vi "Live window-Refresh graphs.vi"(9 "Right Channel":T2, 10 "Left Channel":T2, 11 "Element to queue":T3) -> (0 "Right image":T1, 1 "Enable right image":bool, 2 "Enable left image":bool, 3 "Left image":T1)   [LabVIEW 2013]
uses:
  Queue/Live graphs queue/Typedefs/Live imaging queue element.ctl
  <vilib>/vision/Image Controls.llb/IMAQ Image.ctl
  Typedefs/Channel Selector.ctl
  Typedefs/Left-Right enum.ctl
  Global Variables/gl_UI Ctrl Refs.vi
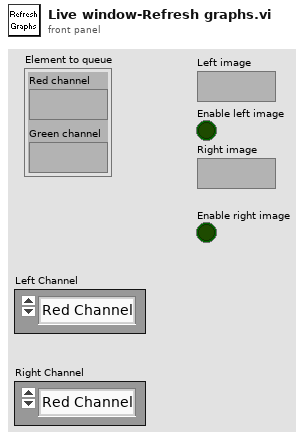
[diagram p1: front panel]
types:
  T1 = typedef "IMAQ Image.ctl" = refnum<image>
  T2 = typedef "Channel Selector.ctl" = enum16{"Red Channel", "Green Channel", "Blended"}
  T3 = typedef "Live imaging queue element.ctl" = cluster{"Red channel":T1, "Green channel":T1}
  T4 = typedef "Left-Right enum.ctl" = enum16{"Right", "Left"}
  T5 = typedef "UI ctrl refs cluster.ctl" = cluster{"Top level VI path":path, "Top level VI ref":refnum<vi>, "User menu ref":refnum<k9>, "Sub Panel control":refnum<vi>, "Imaging Param Tab":refnum<vi>, "Occurrence-Start drivers":refnum<k4>, "Occurrence-Speed logging initialised":refnum<k4>, "Occurrence-XYZ stage initialised":refnum<k4>, "Exit button":refnum<vi>, "Status ind":refnum<vi>, "Return to Origin":refnum<vi>, "Speed Logging":refnum<vi>, "Time Lapse":refnum<vi>, "Live Imaging":refnum<vi>, "AOL Z Stack":refnum<vi>, "Motor Z Stack":refnum<vi>, "Funct Acq button":refnum<vi>, "Hard Shutter":refnum<vi>, "Virtual Shutter":refnum<vi>, "Laser Power":refnum<vi>, "AOL Mode":refnum<vi>, "Frame Size":refnum<vi>, "Field of View":refnum<vi>, "Dwell Time":refnum<vi>, "Zoom":refnum<vi>, "AOL Z":refnum<vi>, "Objective":refnum<vi>, "Axis":refnum<vi>, "Paths & Names":refnum<vi>, "Experiment folder path (ind.)":refnum<vi>, "Last State (Ind.)":refnum<vi>, "Laser wavelength ind (nm)":refnum<vi>, "Averages":refnum<vi>, "Angle (degrees)":refnum<vi>, "X centre":refnum<vi>, "Y centre":refnum<vi>, "Plane Mode":refnum<vi>, "# Planes":refnum<vi>, "Z Start":refnum<vi>, "Z Stop":refnum<vi>, "Z Step":refnum<vi>, "PMT 1":refnum<vi>, "PMT 2":refnum<vi>, "Stage XYZ Position":refnum<vi>, "Pockels@Z Start":refnum<vi>, "Pockels@Z Stop":refnum<vi>, "Obtain Z Start":refnum<vi>, "Obtain Z Stop":refnum<vi>, "Live stim.trig.period":refnum<vi>, "Live stim.trig.enable":refnum<vi>, "Funct. Acq. Pockels Modulation":refnum<vi>, "Enable Video Recording":refnum<vi>, "Video Record-Live Imaging":refnum<vi>, "Video Record-Funct acq":refnum<vi>, "AOL Z-stack Chirps Ready (ind)":refnum<vi>, "Center freq ind (nm)":refnum<vi>, "Logging queue (ind)":refnum<vi>, "Back aperture power (ind.)":refnum<vi>, "Power after objective (ind.)":refnum<vi>, "Switch user":refnum<vi>}
  T6 = typedef "PMT control knob.ctl" = u16
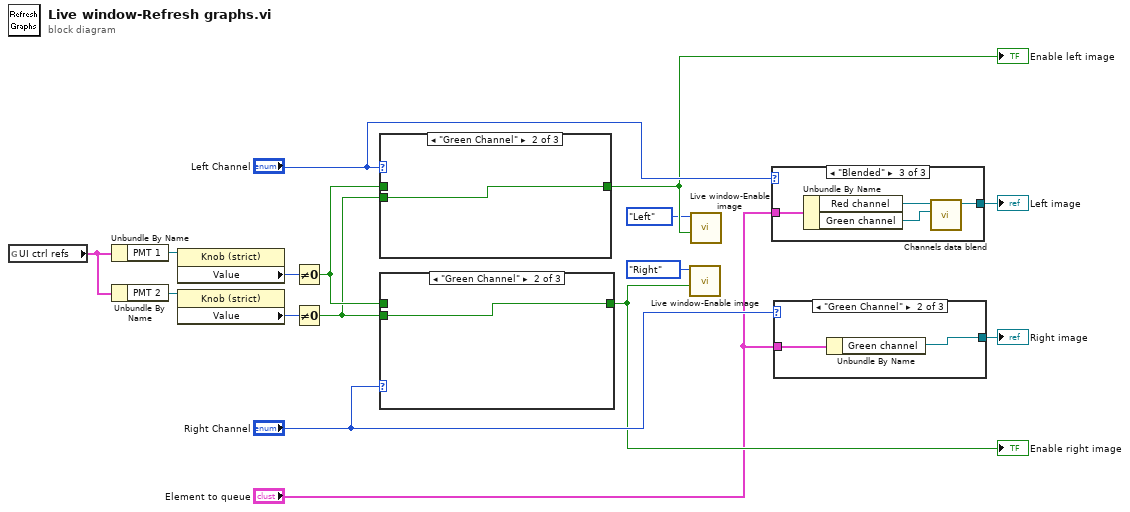
[diagram p0: block diagram]
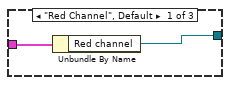
[diagram p2: hidden frame]
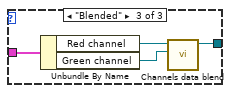
[diagram p3: hidden frame]
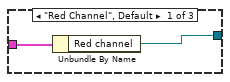
[diagram p4: hidden frame]
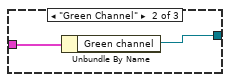
[diagram p5: hidden frame]
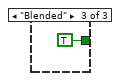
[diagram p7: hidden frame]
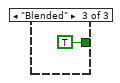
[diagram p9: hidden frame]
diagram:
  n1 = global read "gl_UI Ctrl Refs.vi" "UI ctrl refs"() -> (w12:T5)
  n2 = Unbundle By Name(w12) -> ("PMT 1"=w14:refnum<vi>)
  n3 = Unbundle By Name(w12) -> ("PMT 2"=w13:refnum<vi>)
  n4 = property on="Property Node" class="Knob (strict)"(reference=w14) -> ("Value"=w11:T6)  [unwired: 1 in, 2 out]
  n5 = property on="Property Node" class="Knob (strict)"(reference=w13) -> ("Value"=w10:T6)  [unwired: 1 in, 2 out]
  n6 = Not Equal To 0?(x=w11) -> (x != 0?=w5:bool)
  n7 = Not Equal To 0?(x=w10) -> (x != 0?=w4:bool)
  n8 = case shown="\"Green Channel\"" "Left Channel" {
    tunnel: w5 -> [w17 _ _]
    tunnel: w4 -> [_ w18 _]
    tunnel: [w17 w18 TRUE] -> w9
    frame "Red Channel", Default {
    }
    frame "Green Channel" {
    }
    frame "Blended" {
    }
  }
  "Enable left image" <- w9
  n9 = case shown="\"Green Channel\"" "Right Channel" {
    tunnel: w5 -> [w20 _ _]
    tunnel: w4 -> [_ w21 _]
    tunnel: [w20 w21 TRUE] -> w8
    frame "Red Channel", Default {
    }
    frame "Green Channel" {
    }
    frame "Blended" {
    }
  }
  "Enable right image" <- w8
  n10 = call "Live window-Enable image.vi"("Enable"=w8, "Which image display?"=Left-Right_enum."Right") -> ()  [unwired: 10 in]
  n11 = call "Live window-Enable image.vi"("Enable"=w9, "Which image display?"=Left-Right_enum."Left") -> ()  [unwired: 10 in]
  n12 = case shown="\"Blended\"" "Left Channel" {
    tunnel: "Element to queue" -> [w24 w26 w30]
    tunnel: [w23 w25 w27] -> w6
    frame "Red Channel", Default {
      n13 = Unbundle By Name(w24) -> ("Red channel"=w23:T1)
    }
    frame "Green Channel" {
      n14 = Unbundle By Name(w26) -> ("Green channel"=w25:T1)
    }
    frame "Blended" {
      n15 = Unbundle By Name(w30) -> ("Red channel"=w29:T1, "Green channel"=w28:T1)
      n16 = call "Channels data blend.vi"("GREEN"=w28, "RED"=w29) -> ("Image Out"=w27:T1)  [unwired: 8 in, 1 out]
    }
  }
  "Left image" <- w6
  n17 = case shown="\"Green Channel\"" "Right Channel" {
    tunnel: "Element to queue" -> [w32 w34 w38]
    tunnel: [w31 w33 w35] -> w7
    frame "Red Channel", Default {
      n18 = Unbundle By Name(w32) -> ("Red channel"=w31:T1)
    }
    frame "Green Channel" {
      n19 = Unbundle By Name(w34) -> ("Green channel"=w33:T1)
    }
    frame "Blended" {
      n20 = Unbundle By Name(w38) -> ("Red channel"=w37:T1, "Green channel"=w36:T1)
      n21 = call "Channels data blend.vi"("GREEN"=w36, "RED"=w37) -> ("Image Out"=w35:T1)  [unwired: 8 in, 1 out]
    }
  }
  "Right image" <- w7
